vi "LoadMaskList.vi"(0 "JunctionList":refnum<vi>, 6 "url 2":string, 8 "UiDefinition 2":T1, 9 "url":string, 10 "Masks":string, 11 "Microsites ref":refnum<k24>) -> (1 "body":string, 2 "body 2":string, 3 "Path":path)   [LabVIEW 2020]
uses:
  C:/Users/User/Desktop/Automation/CurrentVersion/LabviewDXFViewer/bin/Release/LabviewDXFViewer.exe
  LabviewDXFViewer/bin/Release/LabviewDXFViewer.exe
  UIReferences.ctl
  <vilib>/httpClient/LabVIEWHTTPClient.lvlib
panel:
  out "error out":errorcluster
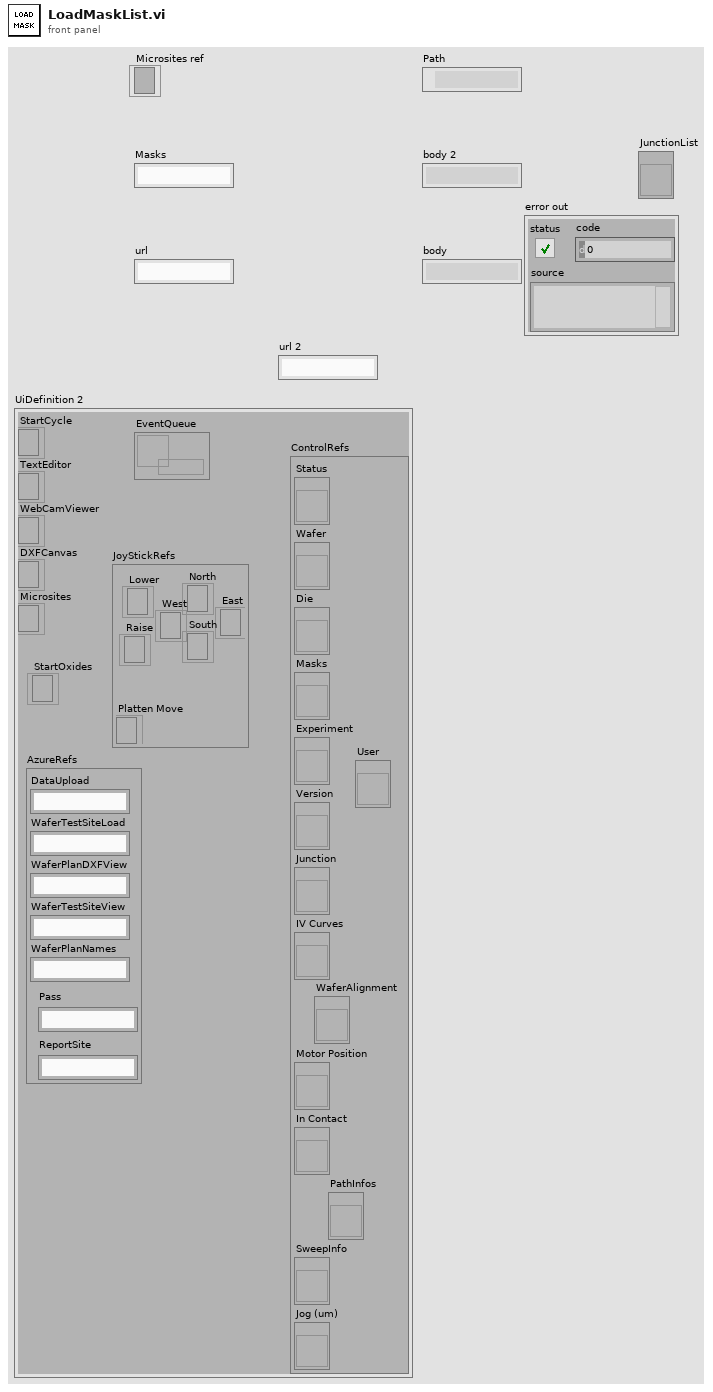
[diagram p1: front panel]
types:
  T1 = typedef "UIReferences.ctl" = cluster{"StartCycle":refnum<k24>, "TextEditor":refnum<k24>, "WebCamViewer":refnum<k24>, "DXFCanvas":refnum<k24>, "Microsites":refnum<k24>, "JoyStickRefs":cluster{"North":refnum<k24>, "Lower":refnum<k24>, "Raise":refnum<k24>, "Platten Move":refnum<k24>, "West":refnum<k24>, "East":refnum<k24>, "South":refnum<k24>}, "AzureRefs":cluster{"DataUpload":string, "WaferTestSiteLoad":string, "WaferPlanDXFView":string, "WaferTestSiteView":string, "WaferPlanNames":string, "Pass":string, "ReportSite":string}, "ControlRefs":cluster{"Status":refnum<vi>, "Wafer":refnum<vi>, "Die":refnum<vi>, "Masks":refnum<vi>, "Experiment":refnum<vi>, "Version":refnum<vi>, "Junction":refnum<vi>, "IV Curves":refnum<vi>, "Motor Position":refnum<vi>, "In Contact":refnum<vi>, "SweepInfo":refnum<vi>, "Jog (um)":refnum<vi>, "PathInfos":refnum<vi>, "User":refnum<vi>, "WaferAlignment":refnum<vi>}, "EventQueue":refnum<queue>, "StartOxides":refnum<k24>}
  T2 = typedef "LabVIEWHTTPClient.lvlib/ClientHandle.ctl" = refnum<k1>
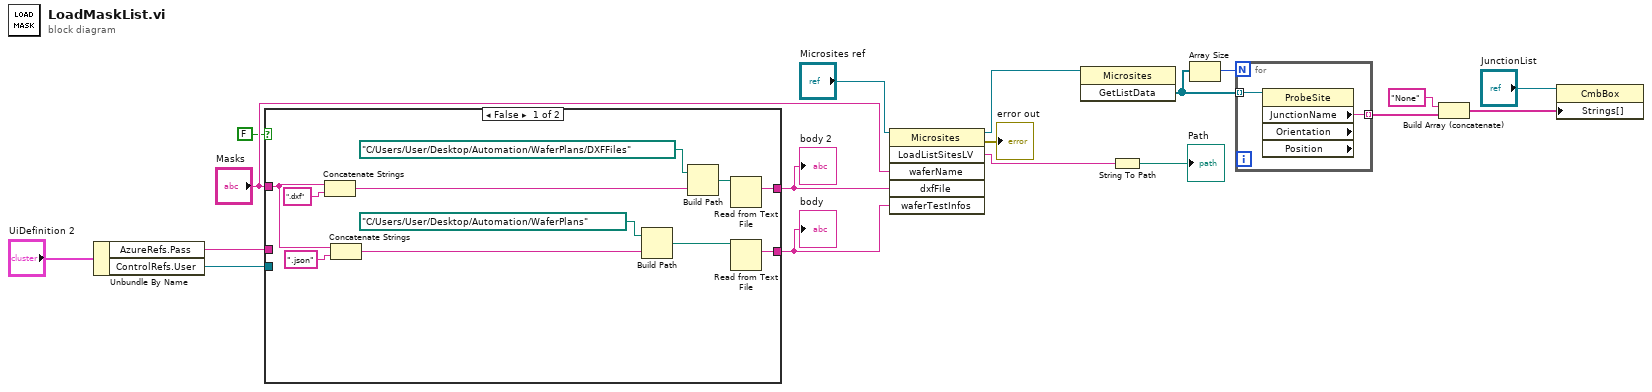
[diagram p0: block diagram]
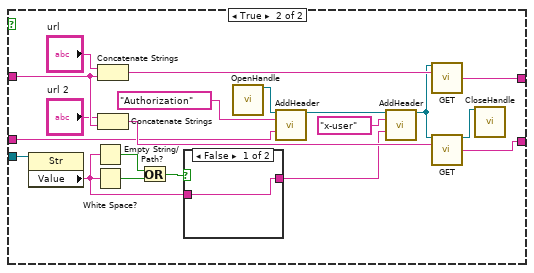
[diagram p2: hidden frame]
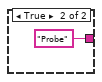
[diagram p3: hidden frame]
diagram:
  n1 = Unbundle By Name("UiDefinition 2") -> ("AzureRefs.Pass"=w3:string, "ControlRefs.User"=w2:refnum<vi>)
  n2 = case shown="False" FALSE {
    tunnel: "Masks" -> [w24 w48]
    tunnel: [w19 w45] -> w15
    tunnel: [w20 w42] -> w14
    tunnel: w3 -> [_ w39]
    tunnel: w2 -> [_ w37]
    frame False {
      n3 = Concatenate Strings(w24, ".dxf" ("string")) -> (w26:string)
      n4 = Concatenate Strings(w24, ".json" ("string")) -> (w22:string)
      n5 = Build Path(base path=path "C:/Users/User/Desktop/Automation/WaferPlans" ("file (use dialog)"), name or relative path=w22) -> (appended path=w21:path)
      n6 = Build Path(base path=path "C:/Users/User/Desktop/Automation/WaferPlans/DXFFiles" ("file (use dialog)"), name or relative path=w26) -> (appended path=w29:path)
      n7 = Read from Text File(file (use dialog)=w29) -> (text=w20:string)  [unwired: 3 in, 3 out]
      n8 = Read from Text File(file (use dialog)=w21) -> (text=w19:string)  [unwired: 3 in, 3 out]
    }
    frame True {
      n9 = property class="Str"(reference=w37) -> ("Value"=w32:string)  [unwired: 1 in, 2 out]
      n10 = Empty String/Path?(string/path=w32) -> (empty?=w33:bool)
      n11 = White Space?(1:w32) -> (0:w36:bool)
      n12 = Concatenate Strings("url", w48) -> (w46:string)
      n13 = Concatenate Strings("url 2", w48) -> (w47:string)
      n14 = Or(x=w33, y=w36) -> (x .or. y?=w34:bool)
      n15 = case shown="False" w34 {
        tunnel: w32 -> [w50 _]
        tunnel: [w50 "Probe"] -> w35
        frame False {
        }
        frame True {
        }
      }
      n16 = call <vilib>:"OpenHandle.vi"() -> ("client handle out"=w31:T2)  [unwired: 14 in, 1 out]
      n17 = call <vilib>:"AddHeader.vi"("client handle"=w31, "header"="Authorization", "value"=w39) -> ("client handle out"=w41:T2)  [unwired: 11 in, 1 out]
      n18 = call <vilib>:"AddHeader.vi"("client handle"=w41, "header"="x-user", "value"=w35) -> ("client handle out"=w30:T2)  [unwired: 11 in, 1 out]
      n19 = call <vilib>:"GET.vi"("client handle"=w30, "url"=w46) -> ("body"=w42:string)  [unwired: 10 in, 3 out]
      n20 = call <vilib>:"GET.vi"("client handle"=w30, "url"=w47) -> ("client handle out"=w43:T2, "body"=w45:string)  [unwired: 10 in, 2 out]
      n21 = call <vilib>:"CloseHandle.vi"("client handle"=w43) -> ()  [unwired: 14 in, 1 out]
    }
  }
  "body" <- w15
  "body 2" <- w14
  n22 = invoke class="Microsites" method="LoadListSitesLV"(reference="Microsites ref", "waferName"="Masks", "dxfFile"=w14, "waferTestInfos"=w15) -> (reference out=w6:refnum<k24>, error out=→"error out":errorcluster, "LoadListSitesLV"=w18:string)  [unwired: 2 in, 3 out]
  n23 = invoke class="Microsites" method="GetListData"(reference=w6) -> ("GetListData"=w12:refnum<k24>[])  [unwired: 2 in, 2 out]
  n24 = String To Path(string=w18) -> (path=→"Path":path)
  n25 = Array Size(array=w12) -> (size(s)=w11:i32)
  n26 = for {
    N: w11 -> [_]
    tunnel: w12 -> [w53] mode=indexing
    tunnel: [w52] -> w10 mode=indexing
    n27 = property class="ProbeSite" props=["JunctionName", "Orientation", "Position"](reference=w53) -> ("JunctionName"=w52:string)  [unwired: 1 in, 4 out]
  }
  n28 = Build Array (concatenate)("None", w10) -> (w8:string[])
  n29 = property class="CmbBox"(reference="JunctionList", "Strings[]"=w8) -> ()  [unwired: 1 in, 2 out]
